vi "Read from Hardware.vi"(8 "error in":errorcluster, 10 "Values in":dbl[](array[numeric]), 11 "Rx UDP Execution Unit in":refnum<class "Rx UDP Execution Unit.lvclass">) -> (0 "error out":errorcluster, 2 "Values out":dbl[](array[numeric]), 3 "Rx UDP Execution Unit out":refnum<class "Rx UDP Execution Unit.lvclass">)   [LabVIEW 2024, in "AIM ARINC 664 Engine.lvlib" / "Implementation.lvlib" / "Rx UDP Execution Unit.lvclass"]
uses:
  Rx UDP Execution Unit.lvclass
  Rx UDP Execution Unit.lvclass/Rx UDP Execution Unit.ctl
  <instrlib>/AIM GmbH/_AIM 664/AIM664LV.lvlib
  <vilib>/Utility/SystemLogging/NI_SystemLogging.lvlib
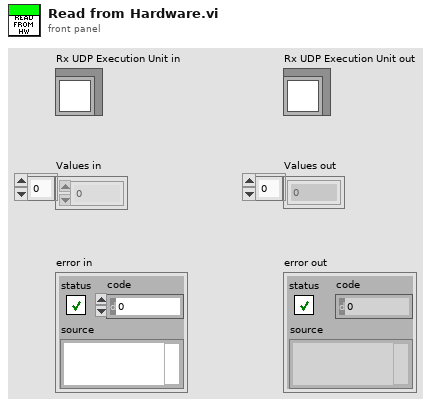
[diagram p1: front panel]
types:
  T1 = typedef "AIM664LV.lvlib/comm_verification_rx.ctl" = cluster{"VlId":u16, "VLRange":u32, "VerificationMode":u32, "Bag":u32, "Jitter":u32, "MaxFrameLength":u32, "MaxSkew":u32, "VLBufSize":u32, "FilterMode":u32, "FilterPosition":u32, "Padding":u32, "FilterMask":u32, "FilterData":u32, "MinFrameLength":u32}
  T2 = typedef "AIM664LV.lvlib/comm_udp_rx.ctl" = cluster{"PortType":enum16{"FDX_UDP_SAMPLING", "FDX_UDP_QUEUING"}, "SubVIId":u32, "domainID":u8, "sideID":u8, "locationID":u8, "partitionID":u8, "UdpSrcPort":u16, "UdpDstPort":u16, "UdpNumBufMessages":u32, "UdpMaxMessageSize":u32, "UdpSamplingRate":u32}
  T3 = cluster{"VL Config":T1, "CommPort Config":T2[]}[]
  T4 = typedef "rx_udp_payload_config.ctl" = cluster{"Data":u8[], "Parameters":cluster{"start index":i32, "size":i32, "encoding":T5, "signed":bool, "scale multiplier":dbl, "scale offset":dbl}[], "GetStatus":bool}
  T5 = typedef "Encoding (Arinc664).ctl" = u16
  T6 = typedef "AIM664LV.lvlib/ReceiveUDPBlockRead.ctl" = cluster{"UDP Handle":u32, "Max Message Size":u32, "Message Buffer":u8[], "UDP Handle Out":u32, "ReadResultCode":i32, "MsgRead":u32}
  T7 = cluster{"start index":i32, "size":i32, "encoding":T5, "signed":bool, "scale multiplier":dbl, "scale offset":dbl}[]
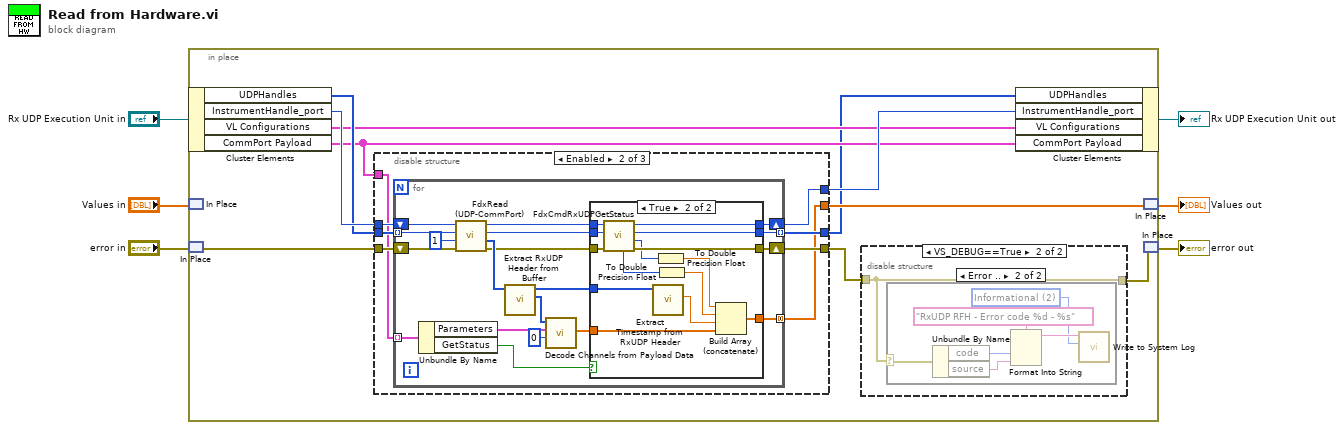
[diagram p0: block diagram]
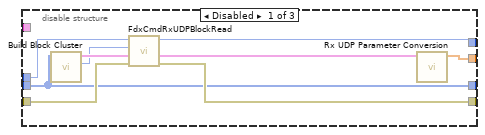
[diagram p4: hidden frame]
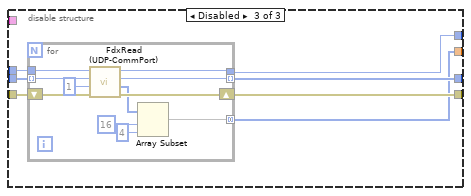
[diagram p6: hidden frame]
diagram:
  n1 = in-place {
    n2 = in-place-cluster #1("Rx UDP Execution Unit in") -> ("UDPHandles"=w13:u32[], "InstrumentHandle_port"=w15:u32, "VL Configurations"=w12:T3, "CommPort Payload"=w11:T4[])
    n3 = in-place-match #2("Values in") -> ()  [unwired: 1 out]
    n4 = in-place-match #3("error in") -> (w16:errorcluster)
    n5 = disable-structure shown="Enabled" {
      disable-tunnel: w16 -> [w33 w38 w82]
      disable-tunnel: [w32 w37 w81] -> w8
      disable-tunnel: w15 -> [w31 w41 w85]
      disable-tunnel: [w30 w40 w84] -> w14
      disable-tunnel: w13 -> [w25 w39 w83]
      disable-tunnel: w11 -> [_ w34 _]
      disable-tunnel: [w26 w35 w79] -> w10
      disable-tunnel: [w25 w36 w80] -> w9
      frame Disabled {
        n6 = call "Build Block Cluster.vi"("UDPHandles in"=w25) -> ("size(s)"=w28:i32, "UDPBlockReadInPorts"=w29:T6[])  [unwired: 9 in]
        n7 = call <instrlib>:"FdxCmdRxUDPBlockRead.vi"("error in"=w33, "RxUDPBlockReadInPortArray"=w29, "PortCountIn"=w28, "InstrumentHandle_port"=w31) -> ("error out"=w32:errorcluster, "RxUDPBlockReadInPortArray"=w27:T6[], "InstrumentHandle_port"=w30:u32)  [unwired: 5 in]
        n8 = call "Rx UDP Parameter Conversion.vi"("RxUDPBlockReadInPortArray"=w27) -> ("Values"=w26:dbl[])  [unwired: 10 in]
      }
      frame Enabled {
        n9 = for {
          tunnel: w39 -> [w59] mode=indexing
          shift-right: [w45] -> w37
          shift-left: w38 -> [w57]
          tunnel: [w43] -> w36 mode=indexing
          tunnel: [w49] -> w35 mode=concatenating
          tunnel: w34 -> [w55] mode=indexing
          shift-right: [w44] -> w40
          shift-left: w41 -> [w60]
          n10 = Unbundle By Name(w55) -> ("Parameters"=w54:T7, "GetStatus"=w42:bool)
          n11 = call <instrlib>:"FdxRead (UDP-CommPort).vi"("error in"=w57, "MsgCount"=u32 1, "UdpHandle"=w59, "InstrumentHandle_port"=w60) -> ("error out"=w46:errorcluster, "ReadBuffer"=w53:u8[], "UdpHandle  Out"=w47:u32, "InstrumentHandle_port"=w48:u32)  [unwired: 3 in, 1 out]
          n12 = call "Extract RxUDP Header from Buffer.vi"("ReadBuffer in"=w53) -> ("Udp Message"=w52:u8[], "Header"=w50:u32[])  [unwired: 9 in]
          n13 = call "Decode Channels from Payload Data.vi"("offset(16)"=0, "Parameters"=w54, "Message Buffer in"=w52) -> ("Channels"=w56:dbl[])  [unwired: 7 in, 1 out]
          n14 = case shown="True" w42 {
            tunnel: w56 -> [w61 w78]
            tunnel: w50 -> [_ w77]
            tunnel: [w61 w76] -> w49
            tunnel: w48 -> [w64 w74]
            tunnel: w47 -> [w63 w73]
            tunnel: w46 -> [w62 w72]
            tunnel: [w62 w71] -> w45
            tunnel: [w64 w70] -> w44
            tunnel: [w63 w69] -> w43
            frame False {
            }
            frame True {
              n15 = call <instrlib>:"FdxCmdRxUDPGetStatus.vi"("error in"=w72, "UdpHandle"=w73, "InstrumentHandle_port"=w74) -> ("error out"=w71:errorcluster, "MsgCount"=w68:u32, "UdpHandle Out"=w69:u32, "InstrumentHandle_port"=w70:u32, "MsgErrorCount"=w66:u32)  [unwired: 4 in]
              n16 = call "Extract Timestamp from RxUDP Header.vi"("header in"=w77) -> ("seconds out"=w75:dbl)  [unwired: 7 in, 3 out]
              n17 = To Double Precision Float(number=w68) -> (double precision float=w67:dbl)
              n18 = To Double Precision Float(number=w66) -> (double precision float=w65:dbl)
              n19 = Build Array (concatenate)(w67, w65, w75, w78) -> (w76:dbl[])
            }
          }
        }
      }
      frame Disabled {
        n20 = for {
          tunnel: w85 -> [w96]
          tunnel: [w95] -> w84
          tunnel: w83 -> [w94] mode=indexing
          shift-right: [w91] -> w81
          shift-left: w82 -> [w92]
          tunnel: [w90] -> w80 mode=indexing
          tunnel: [w88] -> w79 mode=concatenating
          n21 = call <instrlib>:"FdxRead (UDP-CommPort).vi"("error in"=w92, "MsgCount"=u32 1, "UdpHandle"=w94, "InstrumentHandle_port"=w96) -> ("error out"=w91:errorcluster, "ReadBuffer"=w89:u8[], "UdpHandle  Out"=w90:u32, "InstrumentHandle_port"=w95:u32)  [unwired: 3 in, 1 out]
          n22 = Array Subset(array=w89, index=16, length=4) -> (w88:u8[])
        }
      }
    }
    n23 = disable-structure shown="VS_DEBUG==True" {
      disable-tunnel: w8 -> [w17 w18]
      disable-tunnel: [w17 w18] -> w7
      frame condition #0 (active) {
      }
      frame condition #1 {
        n24 = case shown="Error .." w18 {
          selector: w18 -> [_ w19]
          frame No Error {
          }
          frame Error {
            w22 = 2 items=["Error", "Warning", "Informational"] ("severity")
            n25 = Unbundle By Name(w19) -> ("code"=w21:i32, "source"=w20:string)
            n26 = Format Into String(format string="RxUDP RFH - Error code %d - %s", w21, w20) -> (resulting string=w23:string)  [unwired: 2 in, 1 out]
            n27 = call <vilib>:"Write to System Log.vi"("severity"=w22, "message"=w23) -> ()  [unwired: 9 in, 1 out]
          }
        }
      }
    }
    n28 = in-place-cluster #1("UDPHandles"=w9, "InstrumentHandle_port"=w14, "VL Configurations"=w12, "CommPort Payload"=w11) -> (→"Rx UDP Execution Unit out":refnum<class "Rx UDP Execution Unit.lvclass">)
    n29 = in-place-match #2(w10) -> (→"Values out":dbl[])
    n30 = in-place-match #3(w7) -> (→"error out":errorcluster)
  }
